vi "SMART-Moyo (Demo).vi"() -> ()   [LabVIEW 2013]
uses:
  <vilib>/Instr/_visa.llb/VISA Configure Serial Port (Instr).vi
panel:
  out "Compression Depth":dbl(slide) scale=0.0..10.0 scale format="%#_2g"
  out "Compression Rate":dbl(slide) scale=0.0..150.0
  out "Rate 5":bool
  out "Rate 4":bool
  out "Rate 3":bool
  out "Rate 2":bool
  out "Rate":bool
  out "Rate":bool
  out "z-Acceleration":dbl(graph)
  out "subarray 2":dbl[](array[numeric])
  out "Array":dbl[][](array[numeric])
  out "subarray":dbl[](array[numeric])
  out "Sampling Freq. (Hz)":i32=1
  in  "Sample Length (s)":i32(knob)=3 scale=0.0..10.0
  in  "USB Serial Port":refnum<visa-resource-name>="COM4"
  in  "Stop Button":bool
  in  "Start/Stop Training":bool
  # "SMART Moyo"
  # "A low-cost, lightweight CPR mannequin outfitted with inertial sensors that provide real-time feedback"
  # "Controls"
  # "Feedback"
  # "Compression Rate"
  # "Too Slow"
  # "Too Fast"
  # "Compression Depth"
  # "+"
  # "-"
  # "Too Shallow"
  # "Too Deep"
  # "Chris Williams          Last Updated: Apr 28, 2017"
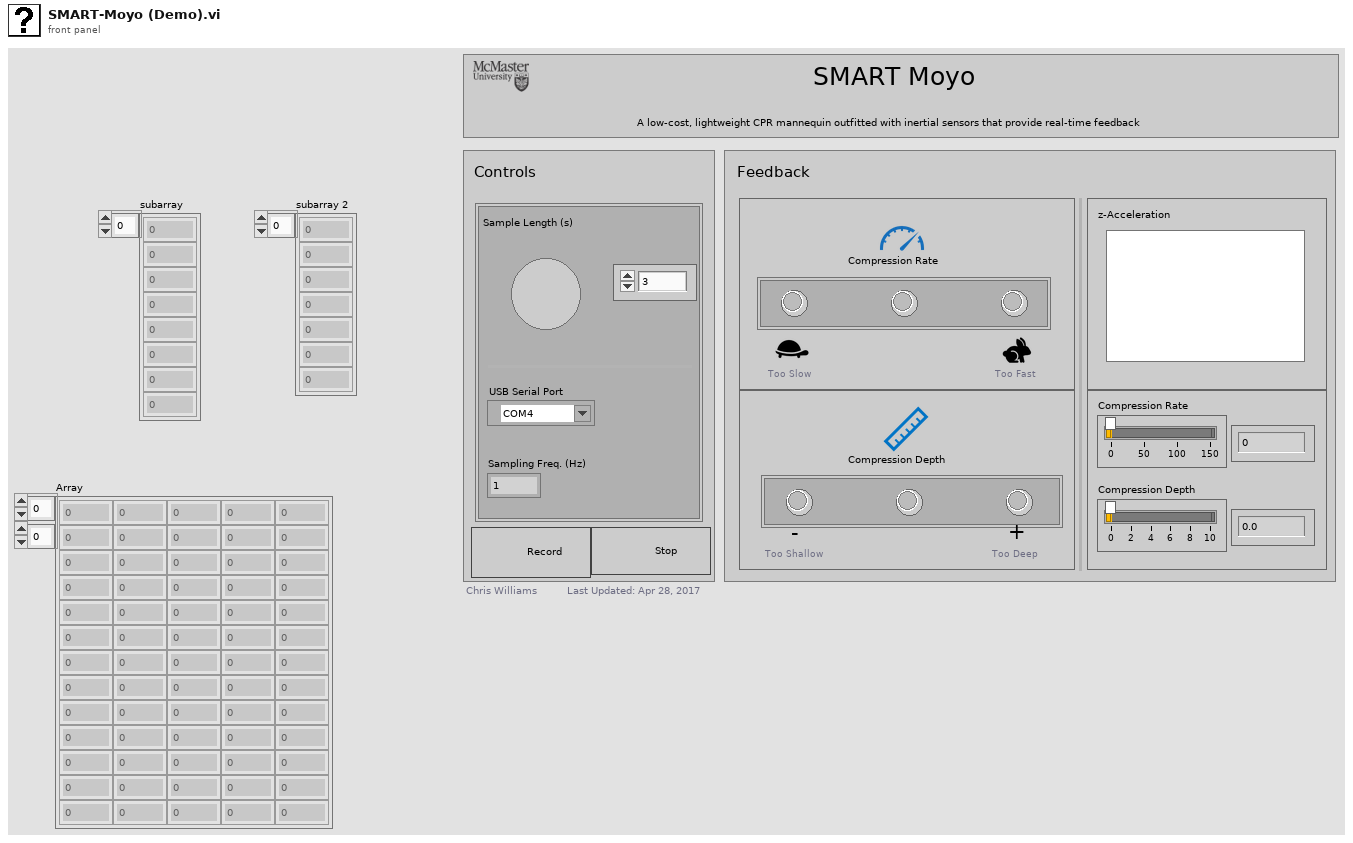
[diagram p1: front panel]
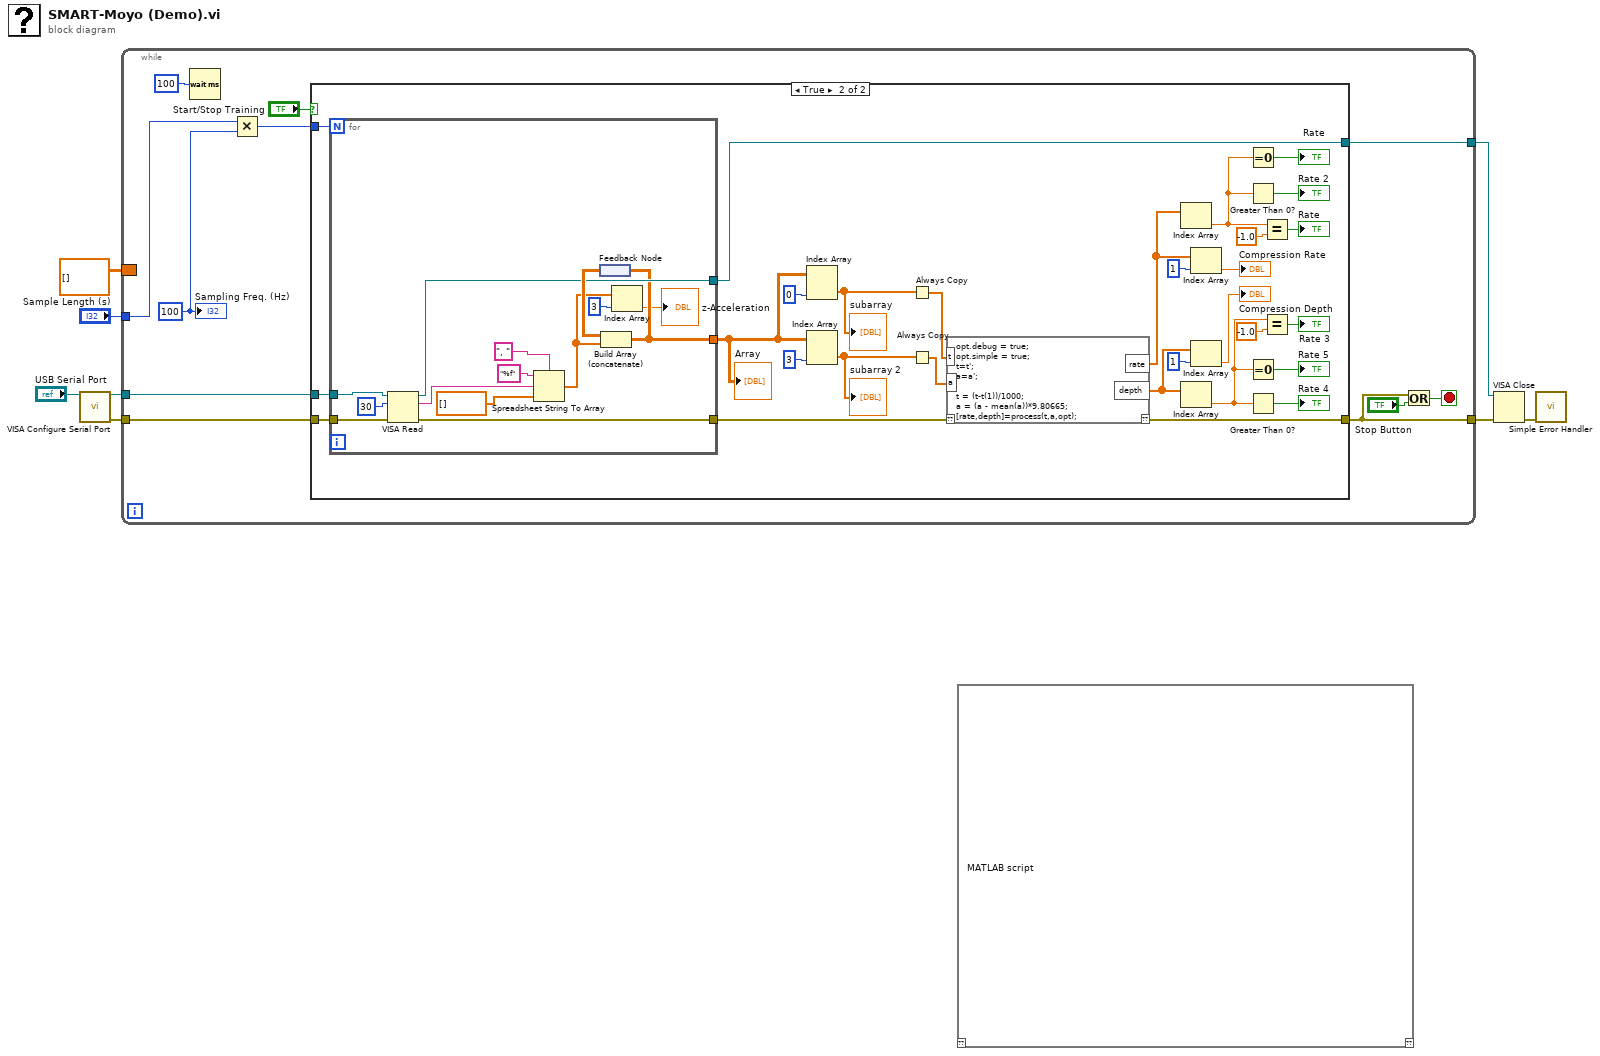
[diagram p0: block diagram]
diagram:
  n1 = call-poly "VISA Configure Serial Port"("VISA resource name"="USB Serial Port") -> ("VISA resource name out"=w4:refnum<visa-resource-name>, "error out"=w3:errorcluster)  [unwired: 13 in]
  n2 = while {
    border: dbl[][] [] -> [_]
    tunnel: [w13] -> w7
    tunnel: w4 -> [w15]
    tunnel: w3 -> [w14]
    tunnel: [w12] -> w2
    tunnel: "Sample Length (s)" -> [w16]
    stop <- w17 stop-if-true
    w9 = 100 ("y")
    n3 = Wait (ms)(milliseconds to wait=u32 100) -> ()  [unwired: 1 out]
    n4 = Multiply(x=w16, y=w9) -> (x*y=w11:i32)
    n5 = case shown="True" "Start/Stop Training" {
      tunnel: w11 -> [_ w50]
      tunnel: w15 -> [w21 w49]
      tunnel: w14 -> [w20 w48]
      tunnel: [w20 w38] -> w13
      tunnel: [w21 w47] -> w12
      frame False {
      }
      frame True {
        n6 = for {
          N: w50 -> [_]
          tunnel: w48 -> [w62]
          tunnel: [w58] -> w39
          tunnel: [w54] -> w45
          tunnel: w49 -> [w63]
          tunnel: [w55] -> w47
          n7 = VISA Read(VISA resource name=w63, byte count=u32 30, error in (no error)=w62) -> (VISA resource name out=w55:refnum<visa-resource-name>, read buffer=w59:string, error out=w58:errorcluster)  [unwired: 1 out]
          n8 = Spreadsheet String To Array(delimiter (Tab)=", ", format string="%f", spreadsheet string=w59, array type (2D Dbl)=dbl[] []) -> (array=w52:dbl[])
          n9 = feedback #1() -> (w56:dbl[][])
          n10 = Build Array (concatenate)(w56, w52) -> (w54:dbl[][])
          n11 = feedback-in #1(w54) -> ()
          n12 = Index Array(array=w52, index=3) -> (element=→"z-Acceleration":dbl)
        }
        "Array" <- w45
        n13 = Index Array(array=w45, index (col)=0 ("disabled index (col)")) -> (element=w43:dbl[])  [unwired: 1 in]
        "subarray" <- w43
        n14 = Index Array(array=w45, index (col)=3 ("disabled index (col)")) -> (element=w41:dbl[])  [unwired: 1 in]
        "subarray 2" <- w41
        n15 = Always Copy(1:w43) -> (0:w42:dbl[])
        n16 = Always Copy(1:w41) -> (0:w40:dbl[])
        n17 = script code="opt.debug = true;\nopt.simple = true;\nt=t';\na=a';\n\nt = (t-t(1))/1000;\na = (a - mean(a))*9.80665;\n[rate,depth]=process(t,a,opt);"("??"=w39, "t"=w42, "a"=w40) -> ("??"=w38:errorcluster, "rate"=w26:dbl[], "depth"=w22:dbl[])
        n18 = Index Array(array=w26) -> (element=w35:dbl)  [unwired: 1 in]
        n19 = Index Array(array=w22) -> (element=w32:dbl)  [unwired: 1 in]
        n20 = Index Array(array=w26, index=1) -> (element=→"Compression Rate":dbl)
        n21 = Index Array(array=w22, index=1) -> (element=→"Compression Depth":dbl)
        n22 = Equal To 0?(x=w35) -> (x = 0?=→"Rate":bool)
        n23 = Greater Than 0?(x=w35) -> (x > 0?=→"Rate 2":bool)
        n24 = Equal To 0?(x=w32) -> (x = 0?=→"Rate 5":bool)
        n25 = Greater Than 0?(x=w32) -> (x > 0?=→"Rate 4":bool)
        n26 = Equal?(x=w35, y=-1.0) -> (x = y?=→"Rate":bool)
        n27 = Equal?(x=w32, y=-1.0) -> (x = y?=→"Rate 3":bool)
      }
    }
    n28 = Or(x=w13, y="Stop Button") -> (x .or. y?=w17:bool)
    "Sampling Freq. (Hz)" <- w9
  }
  n29 = script code="MATLAB script"() -> ()  [unwired: 1 in, 1 out]
  n30 = VISA Close(VISA resource name=w2, error in (no error)=w7) -> (error out=w6:errorcluster)
  n31 = call <vilib>:"Simple Error Handler.vi"("error in (no error)"=w6) -> ()  [unwired: 4 in, 5 out]
